vi "Refresh Knock Listbox.vi"(5 "Knock Listbox Refnum":refnum<vi>, 7 "Knock Sensor Refnum":refnum<vi>, 8 "Knock":u32, 9 "KnockIntensity":sgl[](array[numeric])=[0.0, 0.0, 0.0, 0.0, 0.0, 0.0, 0.0, 0.0, 0.0, 0.0, 0.0, 0.0, 0.0, 0.0, 0.0, 0.0], 10 "CylinderOffsets":sgl[](array[numeric])=[0.0, 0.0, 0.0, 0.0, 0.0, 0.0, 0.0, 0.0, 0.0, 0.0, 0.0, 0.0, 0.0, 0.0, 0.0, 0.0], 11 "SensorSelect":sgl[](array[numeric])=[0.0, 0.0, 0.0, 0.0, 0.0, 0.0, 0.0, 0.0, 0.0, 0.0, 0.0, 0.0, 0.0, 0.0, 0.0, 0.0]) -> ()   [LabVIEW 2016]
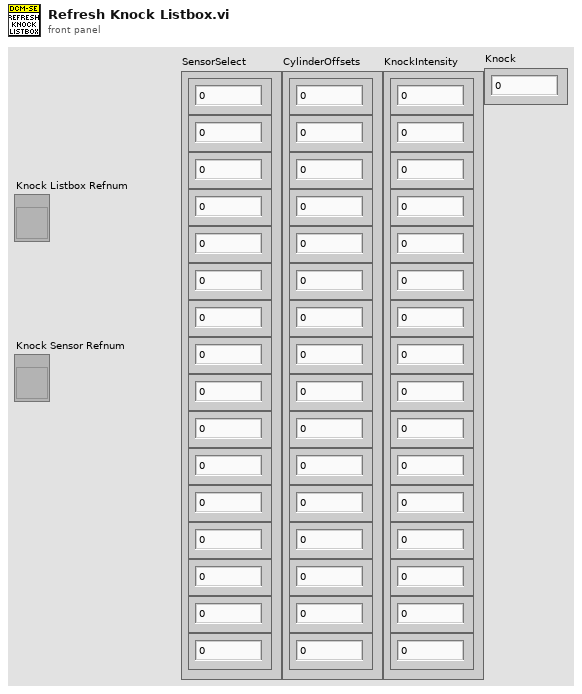
[diagram p1: front panel]
types:
  T1 = typedef "LVStringsAndValuesArrayTypeDef_I32.ctl" = cluster{"String":string, "Value":i32}[]
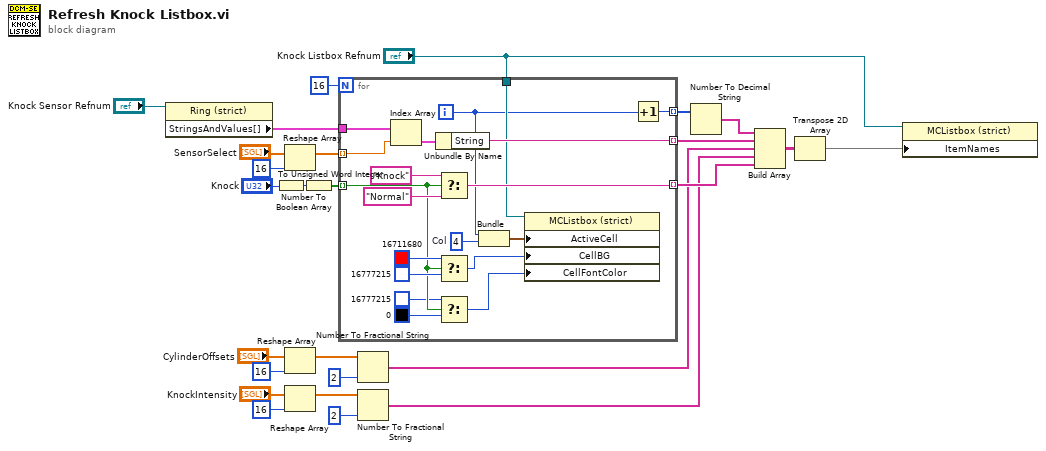
[diagram p0: block diagram]
diagram:
  n1 = property on="Property Node" class="Ring (strict)"(reference="Knock Sensor Refnum") -> ("StringsAndValues[]"=w8:T1)  [unwired: 1 in, 2 out]
  n2 = To Unsigned Word Integer(number="Knock") -> (unsigned 16bit integer=w23:u16)
  n3 = Reshape Array("SensorSelect", 16) -> (w17:sgl[])
  n4 = Reshape Array("CylinderOffsets", 16) -> (w19:sgl[])
  n5 = Reshape Array("KnockIntensity", 16) -> (w21:sgl[])
  n6 = Number To Boolean Array(number=w23) -> (Boolean array=w24:bool[])
  n7 = for {
    N: 16 -> [_]
    tunnel: w8 -> [w45]
    tunnel: w17 -> [w44] mode=indexing
    tunnel: [w42] -> w9 mode=indexing
    tunnel: [w41] -> w11 mode=indexing
    tunnel: w24 -> [w29] mode=indexing
    tunnel: [w38] -> w25 mode=indexing
    tunnel: "Knock Listbox Refnum" -> [w37]
    i -> [w35]
    w36 = 4  # Col
    n8 = Index Array(array=w45, index=w44) -> (element=w43:cluster{"String":string, "Value":i32})
    n9 = Unbundle By Name(w43) -> ("String"=w41:string)
    n10 = Select(t="Knock" ("String"), s=w29, f="Normal" ("String")) -> (s? t:f=w38:string)
    n11 = Select(t=u32 16711680, s=w29, f=u32 16777215) -> (s? t:f=w31:u32)
    n12 = Select(t=u32 16777215, s=w29, f=u32 0) -> (s? t:f=w27:u32)
    n13 = Bundle(w35, "Col"=w36) -> (w34:cluster{i32, "Col":i32})  [unwired: 1 in]
    n14 = property on="Property Node" class="MCListbox (strict)"(reference=w37, "ActiveCell"=w34, "CellBG"=w31, "CellFontColor"=w27) -> ()  [unwired: 1 in, 2 out]
    n15 = Increment(x=w35) -> (x+1=w42:i32)
  }
  n16 = Number To Fractional String(number=w19, precision (6)=i16 2) -> (F-format string=w15:string[])  [unwired: 2 in]
  n17 = Number To Fractional String(number=w21, precision (6)=i16 2) -> (F-format string=w16:string[])  [unwired: 2 in]
  n18 = Number To Decimal String(number=w9) -> (decimal integer string=w10:string[])  [unwired: 1 in]
  n19 = Build Array(w10, w11, w15, w16, w25) -> (w26:string[][])
  n20 = Transpose 2D Array(2D array=w26) -> (transposed array=w2:string[][])
  n21 = property on="Property Node" class="MCListbox (strict)"(reference="Knock Listbox Refnum", "ItemNames"=w2) -> ()  [unwired: 1 in, 2 out]
